vi "FolderMon find changes.vi"(1 "Current File":T3, 2 "All Historic Files":T2(array[cluster])) -> (0 "Changed File":cluster{"File":string, "Change":T1})   [LabVIEW 2011]
uses:
  FolderMon changes.ctl
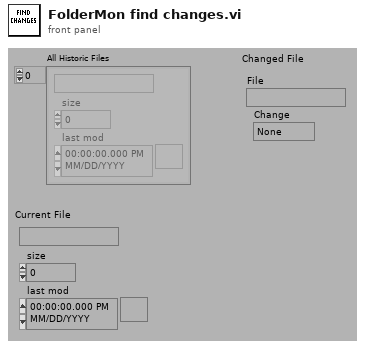
[diagram p1: front panel]
types:
  T1 = typedef "FolderMon changes.ctl" = enum16{"None", "First", "New", "Properties", "Deleted"}
  T2 = cluster{string, "size":i32, "last mod":timestamp}[]
  T3 = cluster{string, "size":i32, "last mod":timestamp}
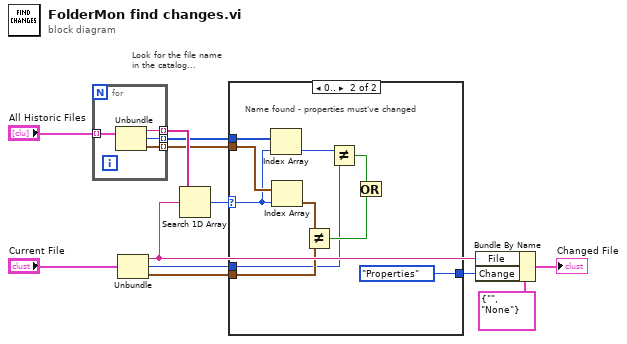
[diagram p0: block diagram]
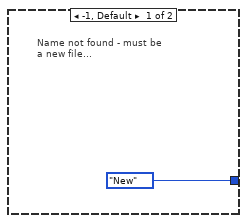
[diagram p2: hidden frame]
diagram:
  # "Look for the file name\nin the catalog..."
  n1 = for {
    tunnel: "All Historic Files" -> [w16] mode=indexing
    tunnel: [w15] -> w10 mode=indexing
    tunnel: [w14] -> w2 mode=indexing
    tunnel: [w13] -> w1 mode=indexing
    n2 = Unbundle(w16) -> (w15:string, "size"=w14:i32, "last mod"=w13:timestamp)
  }
  n3 = Unbundle("Current File") -> (w4:string, "size"=w6:i32, "last mod"=w5:timestamp)
  n4 = Search 1D Array(1D array=w10, element=w4) -> (index of element=w9:i32)  [unwired: 1 out]
  n5 = case shown="0.." w9 {
    selector: w9 -> [_ w25]
    tunnel: w6 -> [_ w20]
    tunnel: w5 -> [_ w24]
    tunnel: [FolderMon_changes."New" ("Change") FolderMon_changes."Properties" ("Change")] -> w3
    tunnel: w2 -> [_ w27]
    tunnel: w1 -> [_ w26]
    frame -1, Default {
      # "Name not found - must be \na new file..."
    }
    frame 0.. {
      # "Name found - properties must've changed"
      n6 = Index Array(array=w27, index=w25) -> (element=w21:i32)
      n7 = Index Array(array=w26, index=w25) -> (element=w23:timestamp)
      n8 = Not Equal?(x=w23, y=w24) -> (x != y?=w22:bool)
      n9 = Not Equal?(x=w21, y=w20) -> (x != y?=w19:bool)
      n10 = Or(x=w19, y=w22) -> ()  [unwired: 1 out]
    }
  }
  n11 = Bundle By Name(cluster=cluster{"File":string, "Change":T1} {"File"="", "Change"=enum."None"} ("Changed File"), "File"=w4, "Change"=w3) -> (→"Changed File":cluster{"File":string, "Change":T1})
